vi "Alpha 2.vi"() -> ()   [LabVIEW 2011]
uses:
  <vilib>/vision/NI_Vision_Development_Module.lvlib
panel:
  in  "Stop":bool
  in  "Browse":bool
  out "Edge":T1(plugin-control)
  in  "Morphology Operation":T2(ring)=enum."Gradient out"
  in  "Threshold Range":cluster{"Lower value":sgl, "Upper value":sgl}={"Lower value"=117.0, "Upper value"=217.0}
  in  "Intensity Color Plane":i32(ring)=7 items=["Red", "Green", "Blue", "Hue", "Saturation", "Luminance", "Value", "Intensity"]
  in  "Image Type":T3 items=["Grayscale (U8)", "Grayscale (I16)", "Grayscale (SGL)", "Complex (CSG)", "RGB (U32)", "HSL (U32)", "RGB (U64)", "Grayscale (U16)"]
  out "Original Image":T1(plugin-control)
  out "Path to Image":path
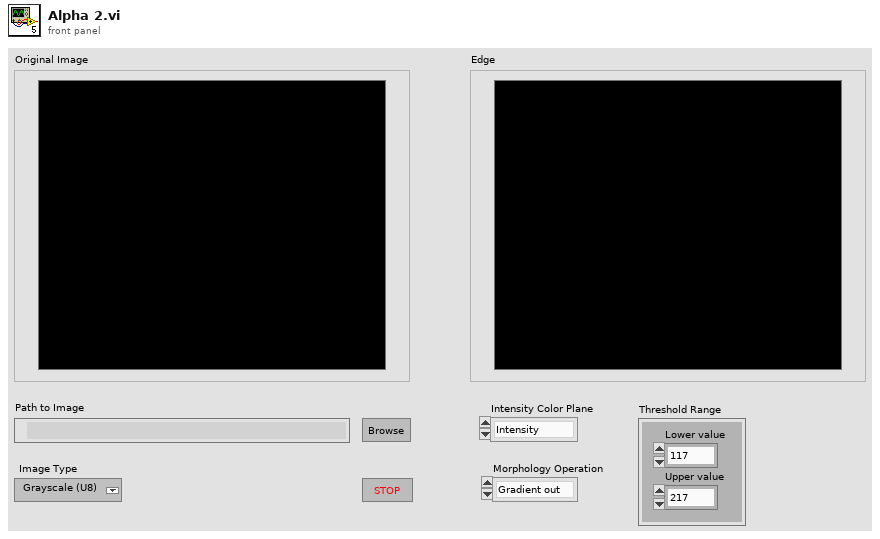
[diagram p1: front panel]
types:
  T1 = typedef "IMAQ Image.ctl" = refnum<image>
  T2 = enum32{"AutoM", "Close", "Dilate", "Erode", "Gradient", "Gradient out", "Gradient in", "Hit miss", "Open", "PClose", "POpen", "Thick", "Thin"}
  T3 = typedef "Image Type" = u32
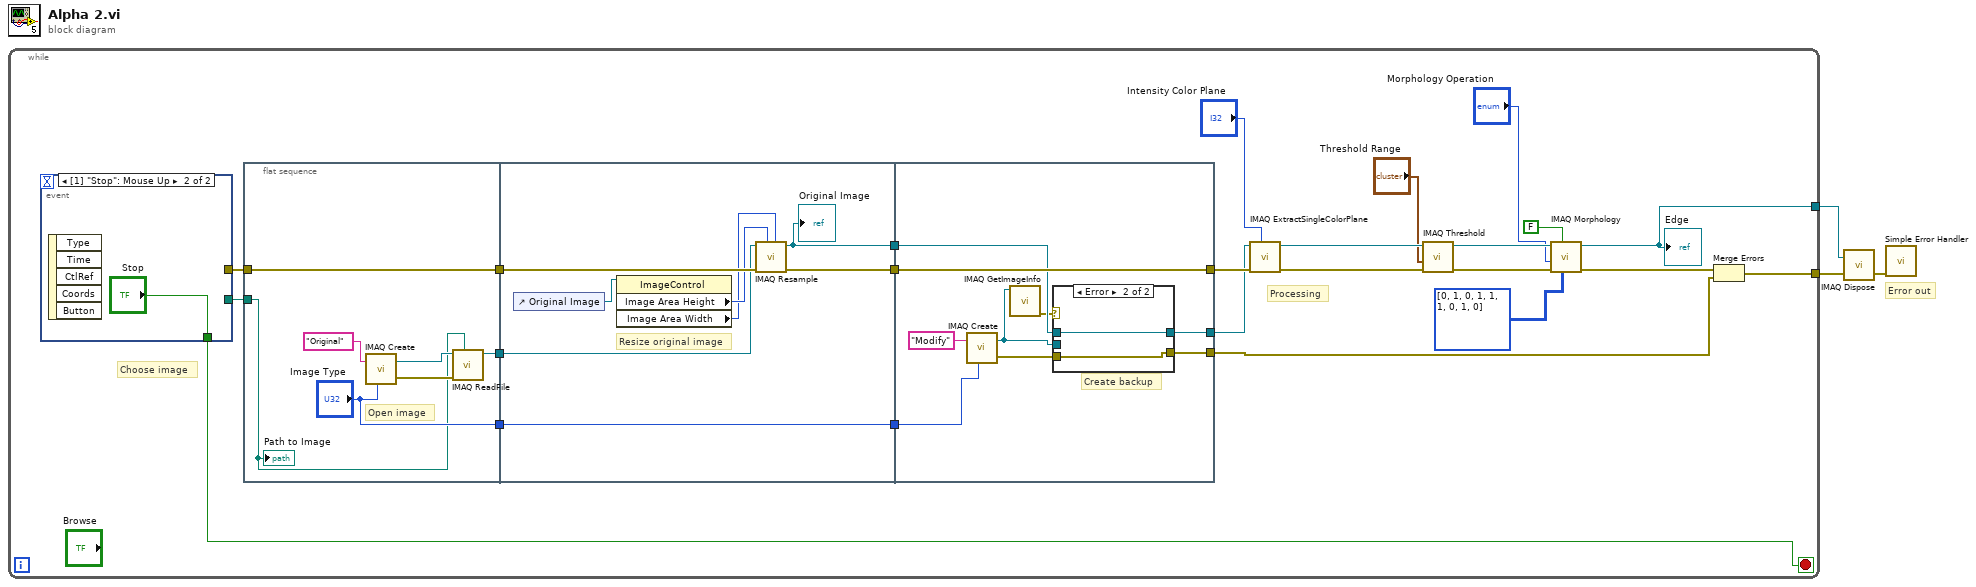
[diagram p0: block diagram]
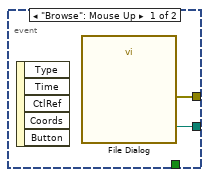
[diagram p2: hidden frame]
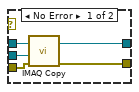
[diagram p3: hidden frame]
diagram:
  # "Error out"
  n1 = while {
    tunnel: [w12] -> w3
    tunnel: [w7] -> w1
    stop <- w4 stop-if-true
    # "Choose image"
    # "Processing"
    n2 = event shown="[1] \"Stop\": Mouse Up" {
      selector: _ -> [_ _]
      dyn-events: _ -> [_ _]
      timeout: _ -> [_ _]
      tunnel: [w29 _] -> w5
      tunnel: [w28 _] -> w6
      tunnel: [_ "Stop"] -> w4
      event "Browse": Mouse Up {
        n3 = event-data() -> ()  [unwired: 1 in, 5 out]
        n4 = call "File Dialog"() -> ("selected path"=w29:path, "error out"=w28:errorcluster)  [unwired: 12 in, 2 out]
      }
      event "Stop": Mouse Up {
        n5 = event-data() -> ()  [unwired: 1 in, 5 out]
      }
    }
    n6 = flat-sequence {
      tunnel: [w32] -> w27
      tunnel: [w34] -> w26
      tunnel: ["Image Type"] -> w25
      tunnel: w6 -> [w32]
      tunnel: w5 -> [w31]
      tunnel: w27 -> [w45]
      tunnel: w26 -> [w44]
      tunnel: [w43] -> w24
      tunnel: [w38] -> w23
      tunnel: [w39] -> w22
      tunnel: w25 -> [w39]
      tunnel: [w54] -> w10
      tunnel: w24 -> [w54]
      tunnel: w23 -> [w48]
      tunnel: [w50] -> w11
      tunnel: [w49] -> w9
      tunnel: w22 -> [w47]
      frame #0 {
        # "Open image"
        n7 = call "IMAQ Create"("Image Name"="Original", "Image Type"="Image Type") -> ("New Image"=w37:T1, "error out"=w36:errorcluster)  [unwired: 3 in]
        n8 = call "IMAQ ReadFile"("File Path"=w31, "error in (no error)"=w36, "Image"=w37) -> ("Image Out"=w34:T1)  [unwired: 4 in, 4 out]
        "Path to Image" <- w31
      }
      frame #1 {
        # "Resize original image"
        n9 = control-ref of="Original Image"() -> (w42:refnum<vi>)
        n10 = property class="ImageControl"(reference=w42) -> ("Image Area Height"=w41:u32, "Image Area Width"=w40:u32)  [unwired: 1 in, 2 out]
        n11 = call "IMAQ Resample"("X Resolution"=w40, "Y Resolution"=w41, "error in (no error)"=w45, "Image Src"=w44) -> ("error out"=w43:errorcluster, "Image Dst Out"=w38:T1)  [unwired: 6 in]
        "Original Image" <- w38
      }
      frame #2 {
        # "Create backup"
        n12 = call "IMAQ Create"("Image Name"="Modify", "Image Type"=w47) -> ("New Image"=w52:T1, "error out"=w53:errorcluster)  [unwired: 3 in]
        n13 = call "IMAQ GetImageInfo"("Image"=w52) -> ("error out"=w46:errorcluster)  [unwired: 1 in, 9 out]
        n14 = case shown="Error" w46 {
          tunnel: w52 -> [w59 _]
          tunnel: [w58 w61] -> w50
          tunnel: [w56 w60] -> w49
          tunnel: w53 -> [w57 w61]
          tunnel: w48 -> [w55 w60]
          frame No Error {
            n15 = call "IMAQ Copy"("error in (no error)"=w57, "Image Dst"=w59, "Image Src"=w55) -> ("error out"=w58:errorcluster, "Image Dst Out"=w56:T1)  [unwired: 3 in]
          }
          frame Error {
          }
        }
      }
    }
    n16 = call "IMAQ ExtractSingleColorPlane"("Color Plane"="Intensity Color Plane", "error in (no error)"=w10, "Image Src"=w9) -> ("error out"=w21:errorcluster, "Image Dst Out"=w20:T1)  [unwired: 1 in, 6 out]
    n17 = call "IMAQ Threshold"("error in (no error)"=w21, "Range"="Threshold Range", "Image Src"=w20) -> ("error out"=w19:errorcluster, "Image Dst Out"=w16:T1)  [unwired: 3 in, 4 out]
    n18 = call "IMAQ Morphology"("Structuring Element"=i32[][] [[0, 1, 0], [1, 1, 1], [0, 1, 0]], "Square/Hexa (Square)"=FALSE, "error in (no error)"=w19, "Operation"="Morphology Operation", "Image Src"=w16) -> ("error out"=w8:errorcluster, "Image Dst Out"=w7:T1)  [unwired: 2 in, 3 out]
    "Edge" <- w7
    n19 = Merge Errors(w8, w11) -> (w12:errorcluster)
  }
  n20 = call "IMAQ Dispose"("Image"=w1, "error in (no error)"=w3) -> ("error out"=w2:errorcluster)  [unwired: 4 in]
  n21 = call <vilib>:"Simple Error Handler.vi"("error in (no error)"=w2) -> ()  [unwired: 4 in, 5 out]
